vi "NI VeriStand - Set Custom Device Channel Faultability.vi"(8 "error in (no error)":errorcluster, 10 "Faultability":bool, 11 "Channel Ref in":T1 format="%.0x") -> (0 "error out":errorcluster, 3 "Channel Ref out":T1=18446744073709551615 format="%.0x")   [LabVIEW 2026, in "Custom Devices Storage.lvlib"]
uses:
  Custom Devices Storage.lvlib
  <vilib>/NI VeriStand/Custom Device API/Custom Device Item Ref.ctl
  C:/Users/Administrator/Desktop/Jatin/All DNC DLLs/NationalInstruments.VeriStand.SystemDefinitionAPI.dll
  Jatin/All DNC DLLs/NationalInstruments.VeriStand.SystemDefinitionAPI.dll
  <vilib>/NI VeriStand/Custom Device API/Custom Device API.lvlib
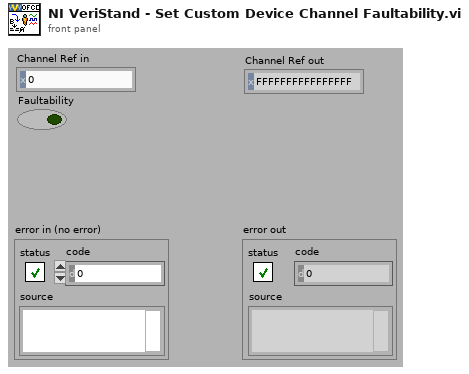
[diagram p1: front panel]
types:
  T1 = typedef "Custom Device API.lvlib/Custom Device Item Ref.ctl" = u64
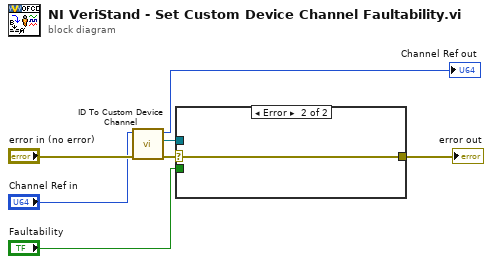
[diagram p0: block diagram]
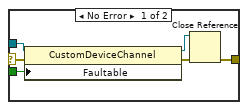
[diagram p2: hidden frame]
diagram:
  n1 = call "ID To Custom Device Channel.vi"("error in (no error)"="error in (no error)", "ID in"="Channel Ref in") -> ("error out"=w6:errorcluster, "NationalInstruments.VeriStand.SystemDefinitionAPI.CustomDeviceChannel"=w7:refnum<k39>, "ID out"=→"Channel Ref out":u64)  [unwired: 7 in]
  n2 = case shown="Error" w6 {
    selector: w6 -> [w11 w14]
    tunnel: w7 -> [w13 _]
    tunnel: "Faultability" -> [w12 _]
    tunnel: [w8 w14] -> w1
    frame No Error {
      n3 = property class="CustomDeviceChannel"(reference=w13, error in=w11, "Faultable"=w12) -> (reference out=w9:refnum<k39>, error out=w10:errorcluster)
      n4 = Close Reference(reference=w9, error in (no error)=w10) -> (error out=w8:errorcluster)
    }
    frame Error {
    }
  }
  "error out" <- w1
